vi "Set Error Status.vi"(8 "error in (no error)":errorcluster, 10 "Sequence":string, 11 "Sequencing in":refnum<class "Sequencing.lvclass">) -> (0 "error out":errorcluster, 3 "Sequencing out":refnum<class "Sequencing.lvclass">)   [LabVIEW 2020, in "VolatusSeq.lvlib" / "Sequencing.lvclass"]
uses:
  Sequencing.lvclass
  Sequencing.lvclass/Sequencing.ctl
  <vilib>/Utility/miscctls.llb/LVMapReplaceAction.ctl
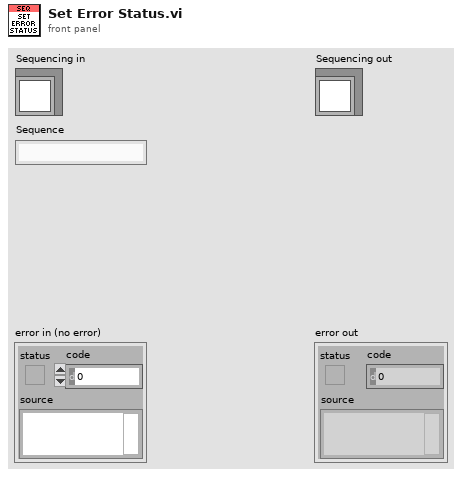
[diagram p1: front panel]
types:
  T1 = typedef "LVMapReplaceAction.ctl" = enum32{"Modify Entry only if found", "Add or Modify Entry", "Delete Entry"}
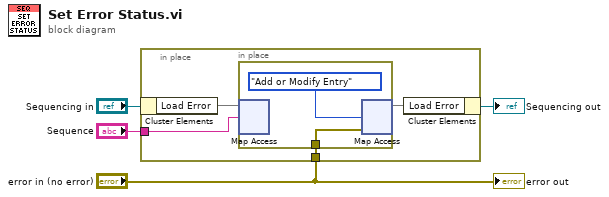
[diagram p0: block diagram]
diagram:
  n1 = in-place {
    in-place-border: "Sequence" -> [w7]
    in-place-border: "error in (no error)" -> [w5]
    n2 = in-place-cluster #1("Sequencing in") -> ("Load Error"=w8:map{string, errorcluster})
    n3 = in-place {
      in-place-border: w5 -> [w9]
      n4 = in-place-map #2(w8, w7) -> ()  [unwired: 1 in, 2 out]
      n5 = in-place-map #2(w9, LVMapReplaceAction."Add or Modify Entry" ("action")) -> (w6:map{string, errorcluster})  [unwired: 2 out]
    }
    n6 = in-place-cluster #1("Load Error"=w6) -> (→"Sequencing out":refnum<class "Sequencing.lvclass">)
  }
  "error out" <- "error in (no error)"
